vi "Set Cell DataType.vi"(8 "error in":errorcluster, 10 "Datatype":i32(ring) items=["Boolean", "Number", "Error", "SharedString", "String", "InlineString", "Date"], 11 "Cell in":refnum<k24>) -> (0 "error out":errorcluster, 3 "Cell out":refnum<k24>)   [LabVIEW 2021, in "Open Xml.lvlib"]
uses:
  Open Xml.lvlib
  D:/git/Open-Xml-LabVIEW/dll/DocumentFormat.OpenXml.dll
  dll/DocumentFormat.OpenXml.dll
  D:/git/Open-Xml-LabVIEW/dll/OpenXmlGenericsWrapper.dll
  dll/OpenXmlGenericsWrapper.dll
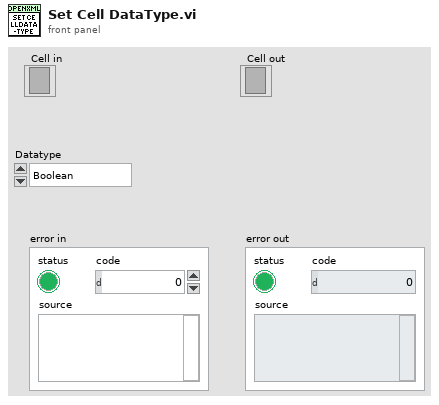
[diagram p1: front panel]
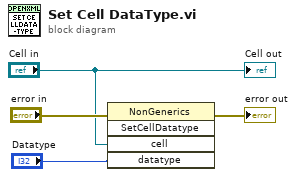
[diagram p0: block diagram]
diagram:
  n1 = invoke class="NonGenerics" method="SetCellDatatype"(error in="error in", "cell"="Cell in", "datatype"="Datatype") -> (error out=→"error out":errorcluster)  [unwired: 2 in, 4 out]
  "Cell out" <- "Cell in"
